vi "status of power_supply1.vi"() -> ()   [LabVIEW 2020]
panel:
  out "status of power_supply1":bool
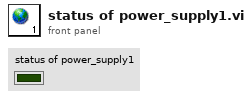
[diagram p1: front panel]
diagram:
